vi "Delete Resource.vi"(8 "error in (no error)":errorcluster, 10 "resource name":string, 11 "Datatype group in":refnum<class "Datatype group.lvclass">) -> (0 "error out":errorcluster, 2 "found":bool, 3 "Datatype group out":refnum<class "Datatype group.lvclass">)   [LabVIEW 2016, in "FPGA RM Shared API.lvlib" / "Datatype group.lvclass"]
uses:
  Datatype group.lvclass
  Datatype group.lvclass/Datatype group.ctl
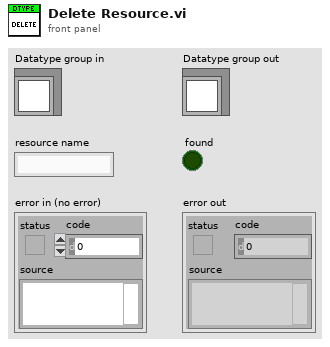
[diagram p1: front panel]
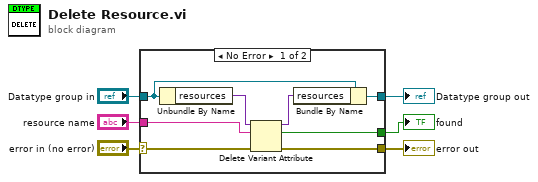
[diagram p0: block diagram]
diagram:
  n1 = case shown="No Error" "error in (no error)" {
    selector: "error in (no error)" -> [w9 w16]
    tunnel: [w8 w16] -> w5
    tunnel: [w14 w15] -> w3
    tunnel: "Datatype group in" -> [w13 w15]
    tunnel: "resource name" -> [w10 _]
    tunnel: [w7 _] -> w1
    frame No Error {
      n2 = Unbundle By Name(w13) -> ("resources"=w12:variant)
      n3 = Delete Variant Attribute(4:w9, 6:w10, 7:w12) -> (0:w8:errorcluster, 2:w7:bool, 3:w11:variant)
      n4 = Bundle By Name(cluster=w13, "resources"=w11) -> (w14:refnum<class "Datatype group.lvclass">)
    }
    frame Error {
    }
  }
  "error out" <- w5
  "Datatype group out" <- w3
  "found" <- w1
